vi "Read Input Registers.vi"(8 "error in (no error)":errorcluster, 9 "number of input registers":u16, 10 "starting address":u16, 11 "Modbus master in":refnum<class "Network Master.lvclass">) -> (0 "error out":errorcluster, 2 "register values":u16[](array[numeric]), 3 "Modbus master out":refnum<class "Network Master.lvclass">)   [LabVIEW 2021, in "Network Master.lvclass"]
doc: "Reads values from contiguous input registers. The maximum number of input registers this VI can read is 125."
uses:
  Network Master.lvclass
  Modbus Data Unit/Modbus Data Unit.lvclass/Modbus Data Unit.ctl
  Network Master.lvclass/Network Master.ctl
  Modbus Data Unit/Construct PDU.vi
  Utility/Bytes to U16s.vi
  Master Function Definition/Function code mismatch error.vi
  Data Model/Error Generator.vi
  Modbus Data Unit/Deconstruct PDU.vi
  Modbus Data Unit/Modbus Data Unit.lvclass
  Transmission Data Unit/Transmission Data Unit.lvclass
  Master Function Definition/Master Function Definition.lvclass
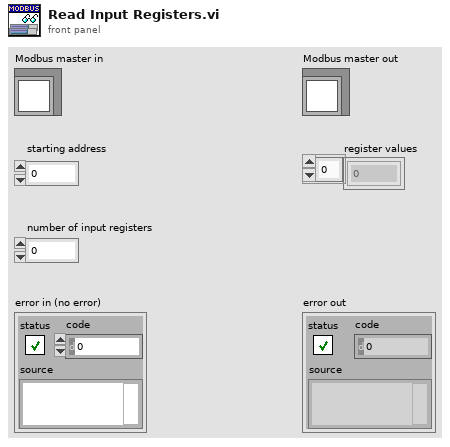
[diagram p1: front panel]
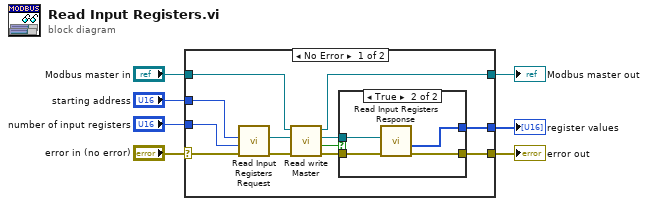
[diagram p0: block diagram]
diagram:
  n1 = case shown="No Error" "error in (no error)" {
    selector: "error in (no error)" -> [w10 w26]
    tunnel: [w17 w26] -> w6
    tunnel: [w9 w25] -> w5
    tunnel: "Modbus master in" -> [w8 w25]
    tunnel: [w16 _] -> w3
    tunnel: "starting address" -> [w15 _]
    tunnel: "number of input registers" -> [w14 _]
    frame No Error {
      n2 = call "Read Input Registers Request.vi"("error in"=w10, "Number of Registers"=w14, "Starting Address"=w15) -> ("error out"=w18:errorcluster, "modbus data unit out"=w11:refnum<class "Modbus Data Unit.lvclass">)  [unwired: 7 in]
      n3 = call "Read write Master.vi"("error in (no error)"=w18, "Modbus data unit in"=w11, "Modbus master in"=w8) -> ("error out"=w19:errorcluster, "PDU valid?"=w13:bool, "Modbus data unit out"=w12:refnum<class "Modbus Data Unit.lvclass">, "Modbus master out"=w9:refnum<class "Network Master.lvclass">)  [unwired: 5 in]
      n4 = case shown="True" w13 {
        tunnel: w19 -> [w20 w24]
        tunnel: [w20 w23] -> w17
        tunnel: w12 -> [_ w22]
        tunnel: [_ w21] -> w16
        frame False {
        }
        frame True {
          n5 = call "Read Input Registers Response.vi"("error in"=w24, "modbus data unit in"=w22) -> ("error out"=w23:errorcluster, "Register Values"=w21:u16[])  [unwired: 7 in, 1 out]
        }
      }
    }
    frame Error {
    }
  }
  "error out" <- w6
  "Modbus master out" <- w5
  "register values" <- w3
